vi "daq_pulsador.vi"() -> ()   [LabVIEW 2011]
panel:
  out "Boolean":bool
  # "El interruptor de tres pines el ground los pines de los lados son el negativo (gnd)y el positivo\nes el de enmedio"
  # "El pulsador de dos pines  un es al gnd i otro al positivo."
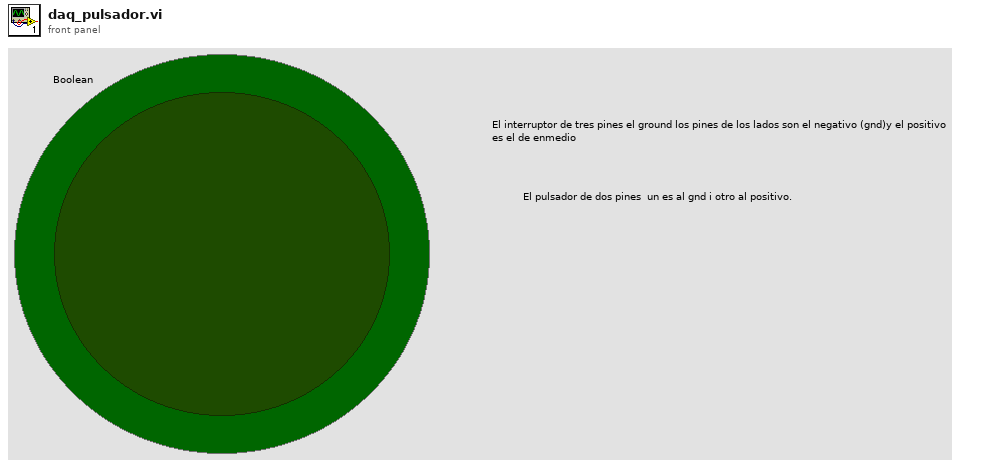
[diagram p1: front panel]
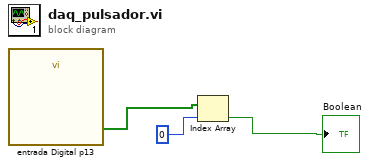
[diagram p0: block diagram]
diagram:
  n1 = call "entrada Digital p13"() -> ("data"=w3:bool[])  [unwired: 17 in, 2 out]
  n2 = Index Array "Index Array"(array=w3, index=0) -> (element=→"Boolean":bool)
